vi "FindLine.vi"(4 "flip interp?":bool, 5 "Box?":bool, 6 "pixels in y":i16=200, 7 "reduce pts by factor of":i32=4, 8 "pixels in x":i16=250, 9 "polar axis":cluster{"r axis":dbl[], "theta axis":dbl[]} {"theta axis" format="%.2f"; "r axis" format="%.2f"}, 10 "Axis scaling Params":T1 {"Y high" format="%.2f"; "Y low" format="%.2f"; "X left" format="%.2f"; "X right" format="%.2f"}, 11 "Sector EndPts":T2 {"y4" format="%.2f"; "x4" format="%.2f"; "y3" format="%.2f"; "x3" format="%.2f"; "y2" format="%.2f"; "x2" format="%.2f"; "y1" format="%.2f"; "x1" format="%.2f"}) -> (0 "sector image line indices":cluster{"x indices":dbl[], "y indices":dbl[]} {"y indices" format="%.2f"; "x indices" format="%.2f"}, 1 "length":i32[](array[numeric]), 2 "y indices":i32[](array[numeric]), 3 "x indices":i32[](array[numeric]))   [LabVIEW 2022 SP3]
uses:
  <vilib>/Analysis/NI_AALBase.lvlib
  <vilib>/Analysis/NI_AALPro.lvlib
panel:
  # "X and Y indices give indices of what was a straight line in the sector format.\nThe length gives the number of RF points starting at X index  along a scan line \n(y index) to form what was a box in the sector ref frame."
  # "These (above) are indices for the sector\nimage (unrounded). The X & Y indices above and to \nthe right are for the \"raw\" rf data image."
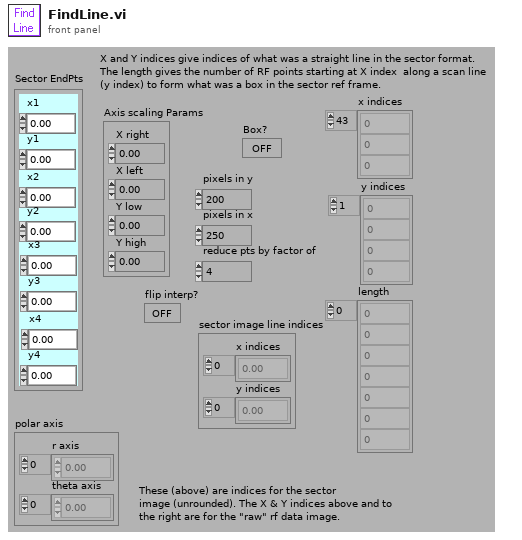
[diagram p1: front panel]
types:
  T1 = cluster{"X right":dbl, "X left":dbl, "Y low":dbl, "Y high":dbl}
  T2 = cluster{"x1":dbl, "y1":dbl, "x2":dbl, "y2":dbl, "x3":dbl, "y3":dbl, "x4":dbl, "y4":dbl}
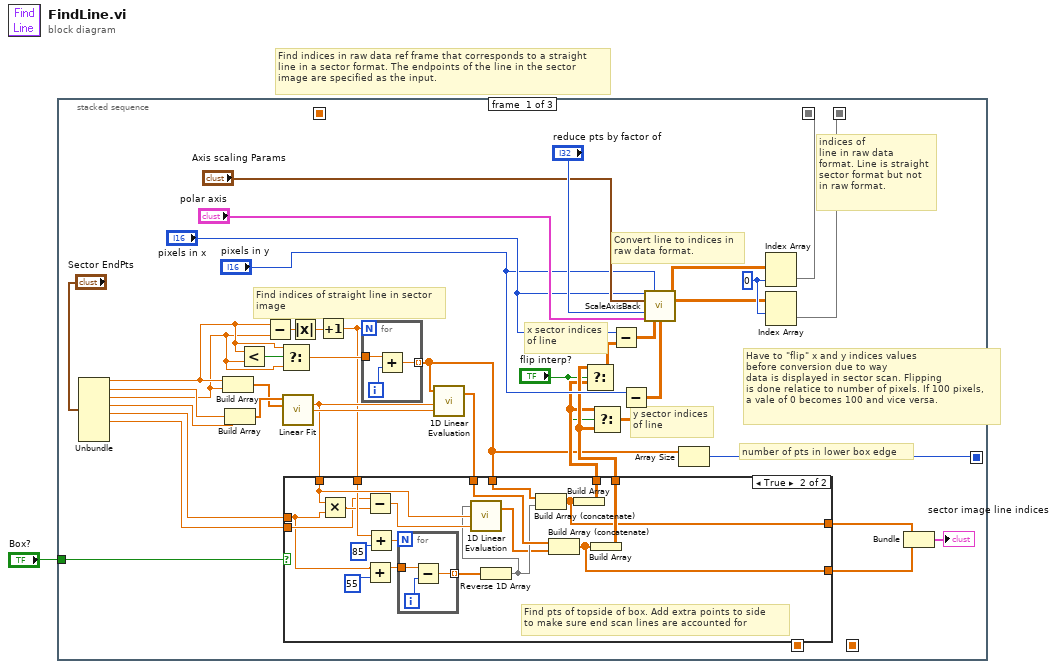
[diagram p0: block diagram]
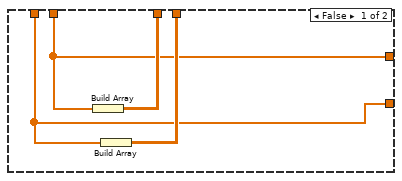
[diagram p2: hidden frame]
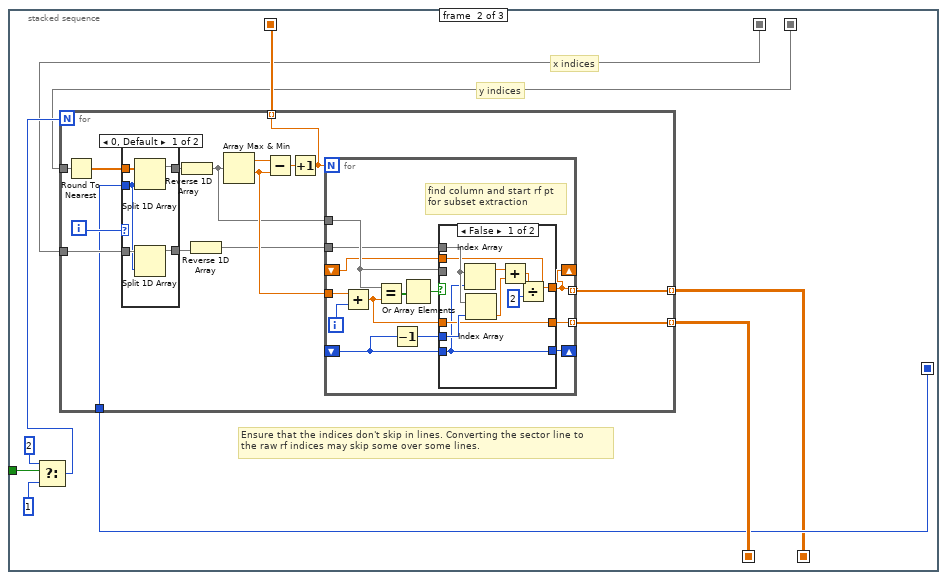
[diagram p3: hidden frame]
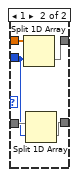
[diagram p4: hidden frame]
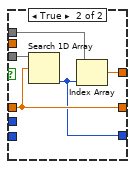
[diagram p5: hidden frame]
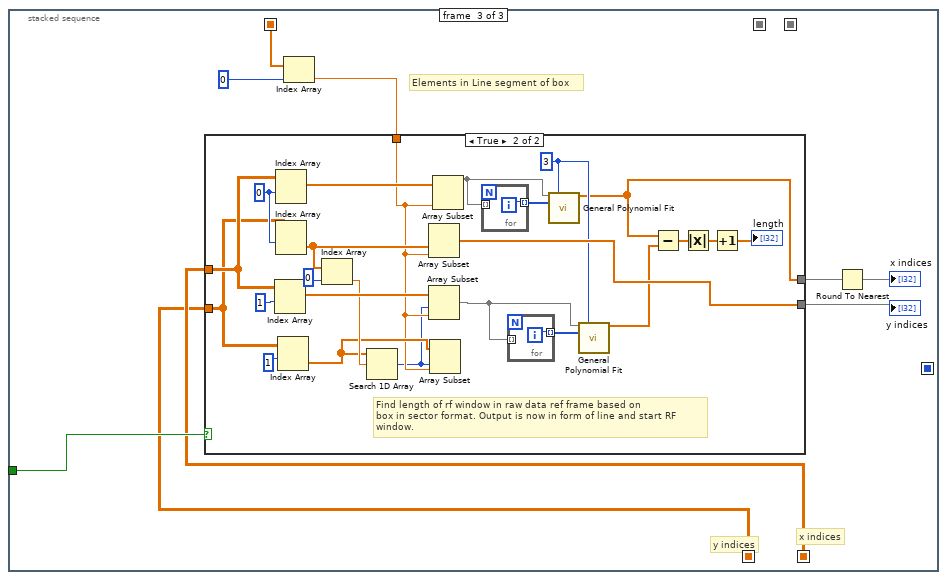
[diagram p6: hidden frame]
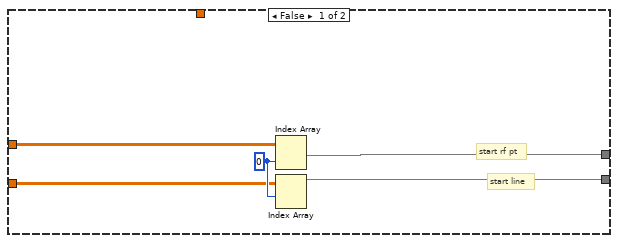
[diagram p7: hidden frame]
diagram:
  # "Find indices in raw data ref frame that corresponds to a straight\nline in a sector format. The endpoints of the line in the sector\nimage are specified as the input."
  n1 = stacked-sequence {
    seq-local: [w27 _ _] -> [_ w72 _]
    seq-local: [w26 _ _] -> [_ w71 _]
    seq-local: [_ w80 _] -> [_ _ w139]
    seq-local: [_ w73 _] -> [_ _ w140]
    seq-local: [_ w79 _] -> [_ _ w137]
    seq-local: [w30 _ _] -> [_ w74 _]
    tunnel: "Box?" -> [w31 w78 w141]
    frame #0 {
      w29 = 0
      # "number of pts in lower box edge"
      # "indices of\nline in raw data\nformat. Line is straight\nsector format but not\nin raw format."
      # "Convert line to indices in\nraw data format."
      # "Find indices of straight line in sector\nimage"
      # "Have to \"flip\" x and y indices values\nbefore conversion due to way\ndata is displayed in sector scan. Flipping\nis done relatice to number of pixels. If 100 pixels,\na vale of 0 becomes 100 and vice versa."
      # "x sector indices\nof line"
      # "y sector indices\nof line"
      n2 = Unbundle("Sector EndPts") -> ("x1"=w23:dbl, "y1"=w22:dbl, "x2"=w21:dbl, "y2"=w20:dbl, "x3"=w19:dbl, "y3"=w18:dbl)  [unwired: 2 out]
      n3 = Build Array(w23, w21) -> (w4:dbl[])
      n4 = Build Array(w22, w20) -> (w5:dbl[])
      n5 = Less?(x=w23, y=w21) -> (x < y?=w39:bool)
      n6 = Subtract(x=w23, y=w21) -> (x-y=w41:dbl)
      n7 = Select(t=w23, s=w39, f=w21) -> (s? t:f=w38:dbl)
      n8 = call <vilib>:"Linear Fit.vi"("Y"=w5, "X"=w4) -> ("slope"=w35:dbl, "intercept"=w37:dbl)  [unwired: 4 in, 8 out]
      n9 = Absolute Value(x=w41) -> (abs(x)=w40:dbl)
      n10 = Increment(x=w40) -> (x+1=w34:dbl)
      n11 = for {
        N: w34 -> [_]
        tunnel: w38 -> [w70]
        tunnel: [w68] -> w3 mode=indexing
        i -> [w69]
        n12 = Add(x=w70, y=w69) -> (x+y=w68:dbl)
      }
      n13 = call <vilib>:"1D Linear Evaluation.vi"("offset"=w37, "scale"=w35, "X"=w3) -> ("Y[i]=X[i]*a+b"=w32:dbl[])  [unwired: 1 out]
      n14 = case shown="True" w31 {
        tunnel: w19 -> [_ w55]
        tunnel: w18 -> [_ w57]
        tunnel: w35 -> [_ w64]
        tunnel: w34 -> [_ w62]
        tunnel: w3 -> [w43 w60]
        tunnel: w32 -> [w42 w59]
        tunnel: [w45 w51] -> w7
        tunnel: [w44 w50] -> w8
        tunnel: [w42 w46] -> w15
        tunnel: [w43 w47] -> w2
        frame False {
          n15 = Build Array(w43) -> (w45:dbl[][])
          n16 = Build Array(w42) -> (w44:dbl[][])
        }
        frame True {
          # "Find pts of topside of box. Add extra points to side\nto make sure end scan lines are accounted for"
          n17 = Multiply(x=w64, y=w55) -> (x*y=w58:dbl)
          n18 = Subtract(x=w57, y=w58) -> (x-y=w63:dbl)
          n19 = Add(x=w55, y=55) -> (x+y=w56:dbl)
          n20 = Add(x=w62, y=85) -> (x+y=w61:dbl)
          n21 = for {
            N: w61 -> [_]
            tunnel: w56 -> [w67]
            tunnel: [w65] -> w52 mode=indexing
            i -> [w66]
            n22 = Subtract(x=w67, y=w66) -> (x-y=w65:dbl)
          }
          n23 = Reverse 1D Array(array=w52) -> (reversed array=w49:dbl[])
          n24 = call <vilib>:"1D Linear Evaluation.vi"("offset"=w63, "scale"=w64, "X"=w49) -> ("Y[i]=X[i]*a+b"=w48:dbl[])  [unwired: 1 out]
          n25 = Build Array (concatenate)(w60, w49) -> (w47:dbl[])
          n26 = Build Array (concatenate)(w59, w48) -> (w46:dbl[])
          n27 = Build Array(w47) -> (w51:dbl[][])
          n28 = Build Array(w46) -> (w50:dbl[][])
        }
      }
      n29 = Select(t=w8, s="flip interp?", f=w7) -> (s? t:f=w10:dbl[][])
      n30 = Select(t=w7, s="flip interp?", f=w8) -> (s? t:f=w9:dbl[][])
      n31 = Subtract(x="pixels in x", y=w10) -> (x-y=w11:dbl[][])
      n32 = Subtract(x="pixels in y", y=w9) -> (x-y=w12:dbl[][])
      n33 = call "ScaleAxisBack.vi"("pixels in x"="pixels in x", "pixels in y"="pixels in y", "Axis scaling Params"="Axis scaling Params", "reduce pts by factor of"="reduce pts by factor of", "polar axis"="polar axis", "x scaled"=w11, "y scaled"=w12) -> ("x indices"=w28:dbl[][], "y indices"=w25:dbl[][])  [unwired: 7 out]
      n34 = Array Size(array=w3) -> (size(s)=w30:i32)
      n35 = Index Array(array=w28, index (row)=w29) -> (element=w27:dbl[])  [unwired: 1 in]
      n36 = Index Array(array=w25, index (row)=w29) -> (element=w26:dbl[])  [unwired: 1 in]
      n37 = Bundle(w2, "Y[i]=X[i]*a+b"=w15) -> (→"sector image line indices":cluster{dbl[], "Y[i]=X[i]*a+b":dbl[]})  [unwired: 1 out]
    }
    frame #1 {
      # "y indices"
      # "x indices"
      # "Ensure that the indices don't skip in lines. Converting the sector line to \nthe raw rf indices may skip some over some lines."
      n38 = Select(t=2, s=w78, f=1) -> (s? t:f=w75:i32)
      n39 = for {
        N: w75 -> [_]
        tunnel: w71 -> [w82]
        tunnel: w72 -> [w89]
        tunnel: [w83] -> w73 mode=indexing
        tunnel: [w92] -> w80 mode=indexing
        tunnel: [w91] -> w79 mode=indexing
        tunnel: w74 -> [w84]
        i -> [w85]
        n40 = Round To Nearest(number=w82) -> (nearest integer value=w81:dbl[])
        n41 = case shown="0, Default" w85 {
          tunnel: w81 -> [w100 w104]
          tunnel: [w97 w105] -> w90
          tunnel: w89 -> [w99 w102]
          tunnel: [w98 w103] -> w88
          tunnel: w84 -> [w96 w101]
          frame 0, Default {
            n42 = Split 1D Array(array=w100, index=w96) -> (first subarray=w97:dbl[])  [unwired: 1 out]
            n43 = Split 1D Array(array=w99, index=w96) -> (first subarray=w98:dbl[])  [unwired: 1 out]
          }
          frame 1 {
            n44 = Split 1D Array(array=w104, index=w101) -> (second subarray=w105:dbl[])  [unwired: 1 out]
            n45 = Split 1D Array(array=w102, index=w101) -> (second subarray=w103:dbl[])  [unwired: 1 out]
          }
        }
        n46 = Reverse 1D Array(array=w90) -> (reversed array=w87:dbl[])
        n47 = Reverse 1D Array(array=w88) -> (reversed array=w86:dbl[])
        n48 = Array Max & Min(array=w87) -> (max value=w95:dbl, min value=w94:dbl)  [unwired: 2 out]
        n49 = Subtract(x=w95, y=w94) -> (x-y=w93:dbl)
        n50 = Increment(x=w93) -> (x+1=w91:dbl)
        n51 = for {
          N: w91 -> [_]
          tunnel: w94 -> [w118]
          tunnel: [w107] -> w83 mode=indexing
          tunnel: [w116] -> w92 mode=indexing
          tunnel: w87 -> [w112]
          tunnel: w86 -> [w108]
          shift-right: [w111] -> _
          shift-left: _ -> [w109]
          shift-right: [w107] -> _
          shift-left: _ -> [w106]
          i -> [w110]
          # "find column and start rf pt\nfor subset extraction"
          n52 = Add(x=w118, y=w110) -> (x+y=w114:dbl)
          n53 = Equal?(x=w112, y=w114) -> (x = y?=w115:bool[])
          n54 = Decrement(x=w109) -> (x-1=w113:i32)
          n55 = Or Array Elements(Boolean array=w115) -> (logical OR=w117:bool)
          n56 = case shown="False" w117 {
            tunnel: w114 -> [w121 w132]
            tunnel: [w119 w131] -> w107
            tunnel: [w121 w132] -> w116
            tunnel: w108 -> [w127 w130]
            tunnel: w112 -> [_ w129]
            tunnel: w109 -> [w120 _]
            tunnel: w113 -> [w126 _]
            tunnel: [w120 w128] -> w111
            tunnel: w106 -> [w119 _]
            frame False {
              n57 = Index Array(array=w127, index=w120) -> (element=w125:dbl)
              n58 = Index Array(array=w127, index=w126) -> (element=w124:dbl)
              n59 = Add(x=w125, y=w124) -> (x+y=w123:dbl)
              n60 = Divide(x=w123, y=2) -> ()  [unwired: 1 out]
            }
            frame True {
              n61 = Search 1D Array(1D array=w129, element=w132) -> (index of element=w128:i32)  [unwired: 1 out]
              n62 = Index Array(array=w130, index=w128) -> (element=w131:dbl)
            }
          }
        }
      }
    }
    frame #2 {
      # "Elements in Line segment of box"
      # "y indices"
      # "x indices"
      n63 = Index Array(array=w137, index=0) -> (element=w136:dbl)
      n64 = case shown="True" w141 {
        tunnel: w140 -> [w145 w158]
        tunnel: w139 -> [w144 w157]
        tunnel: [w143 w147] -> w138
        tunnel: [w142 w152] -> w133
        tunnel: w136 -> [_ w160]
        frame False {
          w146 = 0
          # "start line"
          # "start rf pt"
          n65 = Index Array(array=w145, index (row)=w146) -> (element=w143:dbl[])  [unwired: 1 in]
          n66 = Index Array(array=w144, index (row)=w146) -> (element=w142:dbl[])  [unwired: 1 in]
        }
        frame True {
          w149 = 3 ("polynomial order")
          w170 = 0
          # "Find length of rf window in raw data ref frame based on\nbox in sector format. Output is now in form of line and start RF window."
          n67 = Index Array(array=w158, index (row)=1) -> (element=w164:dbl[])  [unwired: 1 in]
          n68 = Index Array(array=w158, index (row)=w170) -> (element=w166:dbl[])  [unwired: 1 in]
          n69 = Index Array(array=w157, index (row)=w170) -> (element=w165:dbl[])  [unwired: 1 in]
          n70 = Index Array(array=w157, index (row)=1) -> (element=w161:dbl[])  [unwired: 1 in]
          n71 = Index Array(array=w165, index=0) -> (element=w162:dbl)
          n72 = Search 1D Array(1D array=w161, element=w162) -> (index of element=w159:i32)  [unwired: 1 out]
          n73 = Array Subset(array=w165, length=w160) -> (w152:dbl[])  [unwired: 1 in]
          n74 = Array Subset(array=w164, index=w159, length=w160) -> (w151:dbl[])
          n75 = Array Subset(array=w161, index=w159, length=w160) -> ()  [unwired: 1 out]
          n76 = Array Subset(array=w166, length=w160) -> (w148:dbl[])  [unwired: 1 in]
          n77 = for {
            tunnel: w148 -> [_] mode=indexing
            tunnel: [w172] -> w154 mode=indexing
            i -> [w172]
          }
          n78 = for {
            tunnel: [w171] -> w153 mode=indexing
            tunnel: w151 -> [_] mode=indexing
            i -> [w171]
          }
          n79 = call <vilib>:"General Polynomial Fit.vi"("Y"=w148, "polynomial order"=w149, "X"=w154) -> ("Best Polynomial Fit"=w147:dbl[])  [unwired: 9 in, 3 out]
          n80 = call <vilib>:"General Polynomial Fit.vi"("Y"=w151, "polynomial order"=w149, "X"=w153) -> ("Best Polynomial Fit"=w150:dbl[])  [unwired: 9 in, 3 out]
          n81 = Subtract(x=w147, y=w150) -> (x-y=w168:dbl[])
          n82 = Absolute Value(x=w168) -> (abs(x)=w156:dbl[])
          n83 = Increment(x=w156) -> (x+1=→"length":dbl[])
        }
      }
      "y indices" <- w133
      n84 = Round To Nearest(number=w138) -> (nearest integer value=→"x indices":dbl[])
    }
  }
